vi "Get Channel Resistance.vi"(8 "error in (no error)":errorcluster, 10 "Params":variant, 11 "PIPX40 Resistor in":refnum<class "PIPX40 Resistor.lvclass">) -> (0 "error out":errorcluster, 2 "Value":variant, 3 "PIPX40 Resistor out":refnum<class "PIPX40 Resistor.lvclass">)   [LabVIEW 2020, in "Pickering.lvlib" / "PIPX40 Resistor.lvclass"]
uses:
  PIPX40 Resistor.lvclass
  D:/WSGitHub/RTFWK/Realization/PIPX40 Base/PIPX40 Base.lvclass
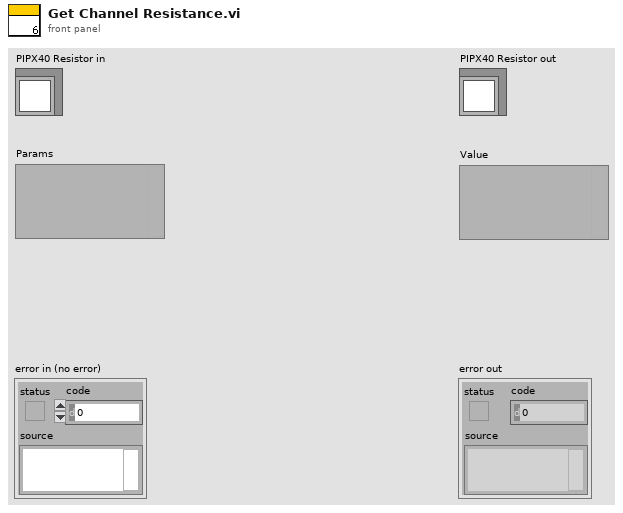
[diagram p1: front panel]
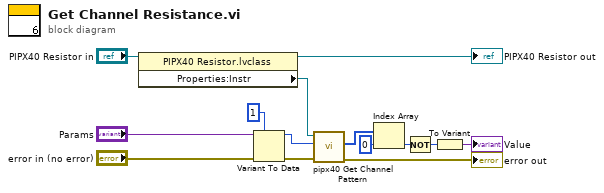
[diagram p0: block diagram]
diagram:
  n1 = property class="PIPX40 Resistor.lvclass"(reference="PIPX40 Resistor in") -> (reference out=→"PIPX40 Resistor out":refnum<class "PIPX40 Resistor.lvclass">, "Properties:Instr"=w7:refnum<visa-resource-name>)  [unwired: 1 in, 1 out]
  n2 = Variant To Data(error in="error in (no error)", type=u32 1 ("subunit number"), Variant="Params") -> (data=w6:u32, error out=w10:errorcluster)
  n3 = call <instrlib>:"pipx40 Get Channel Pattern.vi"("error in (no error)"=w10, "subunit number"=w6, "instrument handle"=w7) -> ("error out"=→"error out":errorcluster, "pattern"=w4:u32[])  [unwired: 6 in, 1 out]
  n4 = Index Array(array=w4, index=0) -> (element=w3:u32)
  n5 = Not(x=w3) -> (.not. x?=w2:u32)
  n6 = To Variant(anything=w2) -> (Variant=→"Value":variant)
